vi "PADMINI_SATO_PRINT_DATA.vi"(7 "SERIAL NO":string, 8 "error in (no error)":errorcluster, 9 "DATE CODE":string, 10 "BRP PART NO":string="NB110460ZA210700L27K1234", 11 "BBI PART NO":string="NB110460ZA210700L27K1234") -> (0 "error out":errorcluster, 2 "SATO BARCODE":string, 3 "result string":string)   [LabVIEW 2017]
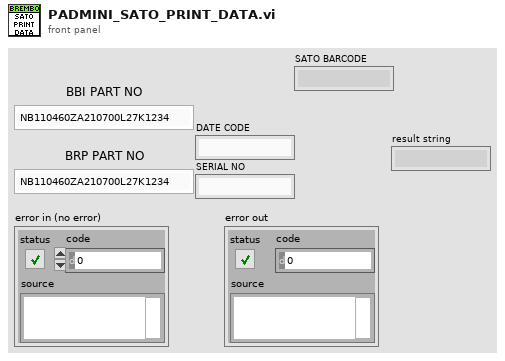
[diagram p1: front panel]
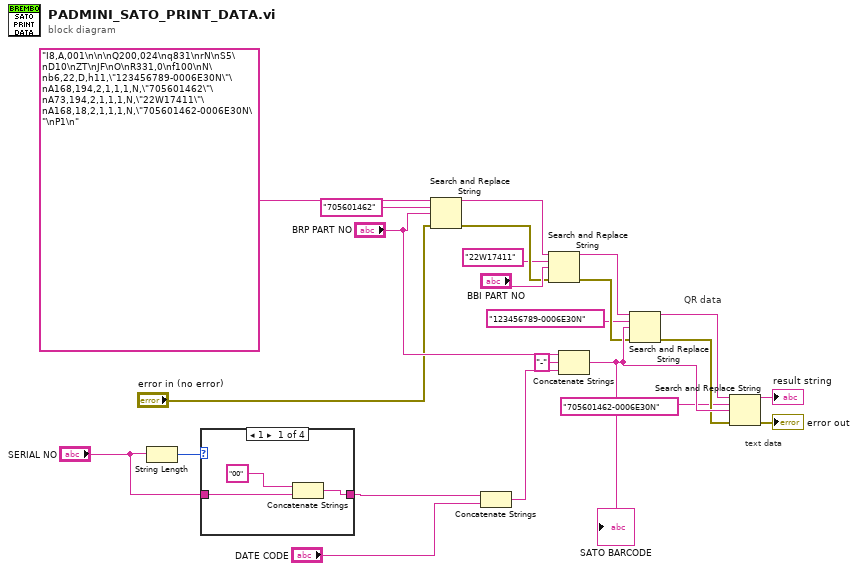
[diagram p0: block diagram]
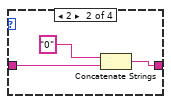
[diagram p2: hidden frame]
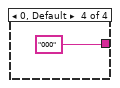
[diagram p4: hidden frame]
diagram:
  # "text data"
  # "QR data"
  n1 = String Length(string="SERIAL NO") -> (length=w3:i32)
  n2 = case shown="1" w3 {
    tunnel: [w24 w27 w30 "000"] -> w1
    tunnel: "SERIAL NO" -> [w25 w28 w30 _]
    frame 1 {
      n3 = Concatenate Strings("00", w25) -> (w24:string)
    }
    frame 2 {
      n4 = Concatenate Strings("0", w28) -> (w27:string)
    }
    frame 3 {
    }
    frame 0, Default {
    }
  }
  n5 = Search and Replace String(input string="I8,A,001\n\n\nQ200,024\nq831\nrN\nS5\nD10\nZT\nJF\nO\nR331,0\nf100\nN\nb6,22,D,h11,\"123456789-0006E30N\"\nA168,194,2,1,1,1,N,\"705601462\"\nA73,194,2,1,1,1,N,\"22W17411\"\nA168,18,2,1,1,1,N,\"705601462-0006E30N\"\nP1\n", search string="705601462", replace string="BRP PART NO", error in="error in (no error)") -> (result string=w8:string, error out=w13:errorcluster)  [unwired: 4 in, 2 out]
  n6 = Concatenate Strings(w1, "DATE CODE") -> (w4:string)
  n7 = Search and Replace String(input string=w8, search string="22W17411", replace string="BBI PART NO", error in=w13) -> (result string=w11:string, error out=w12:errorcluster)  [unwired: 4 in, 2 out]
  n8 = Concatenate Strings("BRP PART NO", "-" ("string"), w4) -> (w21:string)
  "SATO BARCODE" <- w21
  n9 = Search and Replace String(input string=w11, search string="123456789-0006E30N", replace string=w21, error in=w12) -> (result string=w19:string, error out=w20:errorcluster)  [unwired: 4 in, 2 out]
  n10 = Search and Replace String(input string=w19, search string="705601462-0006E30N", replace string=w21, error in=w20) -> (result string=→"result string":string, error out=→"error out":errorcluster)  [unwired: 4 in, 2 out]
